vi "doc_get_subtable_item.vi"(7 "subtables":string[](array[string]), 8 "error in (no error)":errorcluster, 9 "subkeys":string[](array[string]), 11 "toml in":refnum<class "toml.lvclass">) -> (0 "error out":errorcluster, 1 "item (value)":refnum<class "Item.lvclass">, 3 "toml out":refnum<class "toml.lvclass">, 4 "found?":bool)   [LabVIEW 2020, in "toml.lvclass"]
uses:
  toml.lvclass
  Item/Item.lvclass
  toml.lvclass/toml.ctl
  Doc/Doc.lvclass
  Table/Table.lvclass
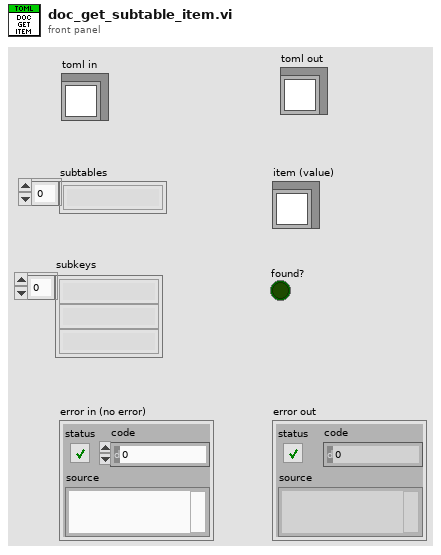
[diagram p1: front panel]
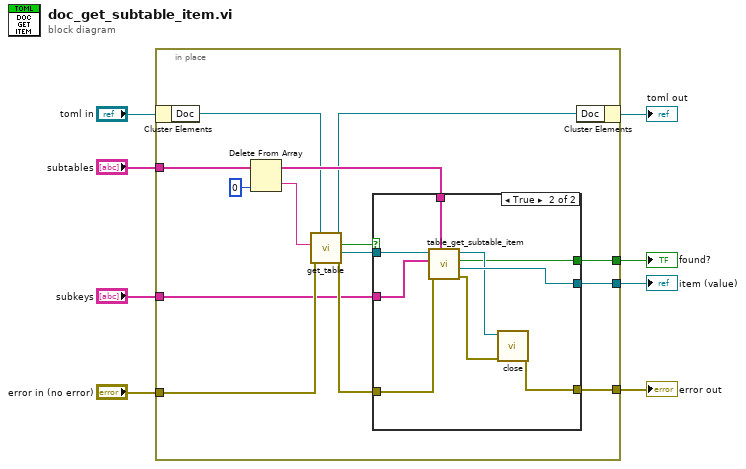
[diagram p0: block diagram]
diagram:
  n1 = in-place {
    in-place-border: [w19] -> w8
    in-place-border: "subtables" -> [w17]
    in-place-border: "error in (no error)" -> [w16]
    in-place-border: "subkeys" -> [w15]
    in-place-border: [w13] -> w4
    in-place-border: [w12] -> w3
    n2 = in-place-cluster #1("toml in") -> ("Doc"=w10:refnum<class "Doc.lvclass">)
    n3 = Delete From Array(array=w17, index=0) -> (deleted portion=w20:string, array with subset deleted=w22:string[])  [unwired: 1 in]
    n4 = call "get_table.vi"("error in (no error)"=w16, "table_name"=w20, "Doc in"=w10) -> ("error out"=w18:errorcluster, "Table"=w14:refnum<class "Table.lvclass">, "found?"=w11:bool, "Doc out"=w9:refnum<class "Doc.lvclass">)  [unwired: 5 in]
    n5 = case shown="True" w11 {
      tunnel: w22 -> [_ w32]
      tunnel: [_ w31] -> w19
      tunnel: w18 -> [w23 w30]
      tunnel: w15 -> [_ w29]
      tunnel: w14 -> [_ w28]
      tunnel: [w23 w25] -> w13
      tunnel: [_ w24] -> w12
      frame False {
      }
      frame True {
        n6 = call "table_get_subtable_item.vi"("subtables"=w32, "error in (no error)"=w30, "subkeys"=w29, "Table in"=w28) -> ("error out"=w26:errorcluster, "item (value)"=w31:refnum<class "Item.lvclass">, "found?"=w24:bool, "Table out"=w27:refnum<class "Table.lvclass">)  [unwired: 4 in]
        n7 = call "close.vi"("error in (no error)"=w26, "Table in"=w27) -> ("error out"=w25:errorcluster)  [unwired: 9 in]
      }
    }
    n8 = in-place-cluster #1("Doc"=w9) -> (→"toml out":refnum<class "toml.lvclass">)
  }
  "error out" <- w4
  "item (value)" <- w8
  "found?" <- w3
